vi "MDAQ_SaveSpectrum.vi"(8 "error in":errorcluster, 10 "Input Array":u32[](array[numeric])) -> (0 "error out":errorcluster)   [LabVIEW 2021]
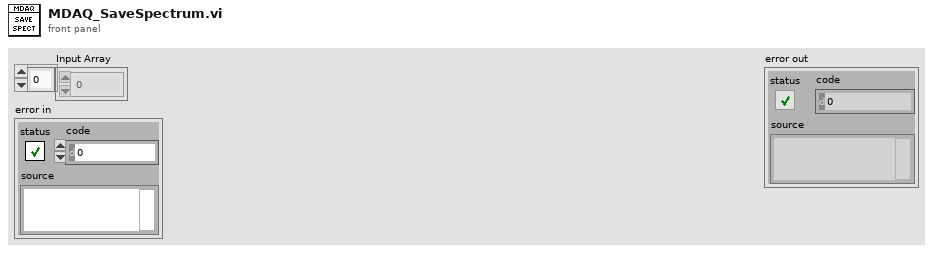
[diagram p1: front panel]
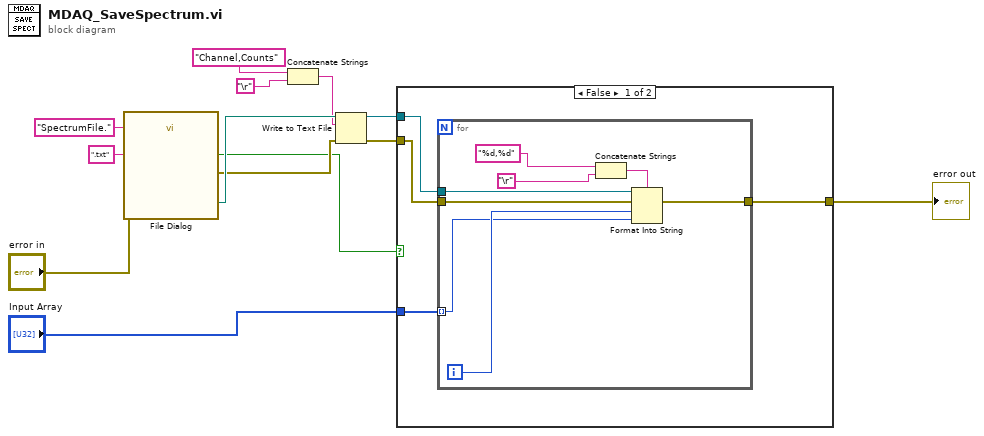
[diagram p0: block diagram]
diagram:
  n1 = call "File Dialog"("default name"="SpectrumFile.", "error in"="error in", "pattern label"=".txt") -> ("selected path"=w11:path, "cancelled"=w6:bool, "error out"=w7:errorcluster)  [unwired: 9 in, 1 out]
  n2 = Concatenate Strings("Channel,Counts" ("text"), "\r") -> (w9:string)
  n3 = Write to Text File(file (use dialog)=w11, text=w9, error in=w7) -> (refnum out=w5:refnum<file>, error out=w4:errorcluster)  [unwired: 1 in, 1 out]
  n4 = case shown="False" w6 {
    tunnel: w5 -> [w16 _]
    tunnel: w4 -> [w15 w26]
    tunnel: "Input Array" -> [w17 _]
    tunnel: [w14 w26] -> w2
    frame False {
      n5 = for {
        tunnel: w17 -> [w24] mode=indexing
        tunnel: w16 -> [w23]
        tunnel: w15 -> [w22]
        tunnel: [w18] -> w14
        i -> [w25]
        n6 = Concatenate Strings("%d,%d" ("format string"), "\r") -> (w21:string)
        n7 = Format Into String(format string=w21, initial string=w23, error in=w22, w25, w24) -> (error out=w18:errorcluster)  [unwired: 1 out]
      }
    }
    frame True {
    }
  }
  "error out" <- w2
